vi "Run.vi"(9 "Team in":refnum<class "Team.lvclass">, 11 "Square in":refnum<class "Square.lvclass">) -> (1 "Team out":refnum<class "Team.lvclass">, 2 "Run Result":T1, 3 "Square out":refnum<class "Square.lvclass">)   [LabVIEW 2020, in "SquareBattle.lvlib" / "Square.lvclass"]
doc: "This VI is called on every active square each turn of the game for the square to decide what action to take.s"
uses:
  Square.lvclass
  Run Result.ctl
  Action.ctl
  Direction.ctl
  Team/Team.lvclass
  Square.lvclass/Square.ctl
  SquareBattle.lvlib
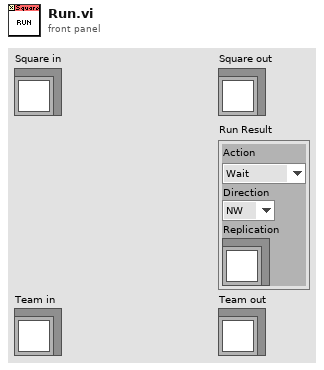
[diagram p1: front panel]
types:
  T1 = typedef "SquareBattle.lvlib/Run Result.ctl" = cluster{"Action":T2, "Direction":T3, "Replication":refnum<class "Square.lvclass">}
  T2 = typedef "SquareBattle.lvlib/Action.ctl" = enum16{"Wait", "Move", "Attack", "Replicate"}
  T3 = typedef "SquareBattle.lvlib/Direction.ctl" = enum16{"NW", "N", "NE", "E", "SE", "S", "SW", "W"}
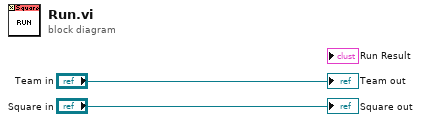
[diagram p0: block diagram]
diagram:
  "Square out" <- "Square in"
  "Team out" <- "Team in"
